vi "Allign Images.vi"(11 "subject file":path) -> (0 "shift":cluster{"left":i16, "top":i16}, 3 "picture":picture)   [LabVIEW 2013]
panel:
  in  "s":bool
  out "Intensity Graph":i16[][](graph)
  out "Array":dbl[](array[numeric])
  out "Master Picture":picture
  out "% matches":dbl
  out "max":i32
  out "rect":T1
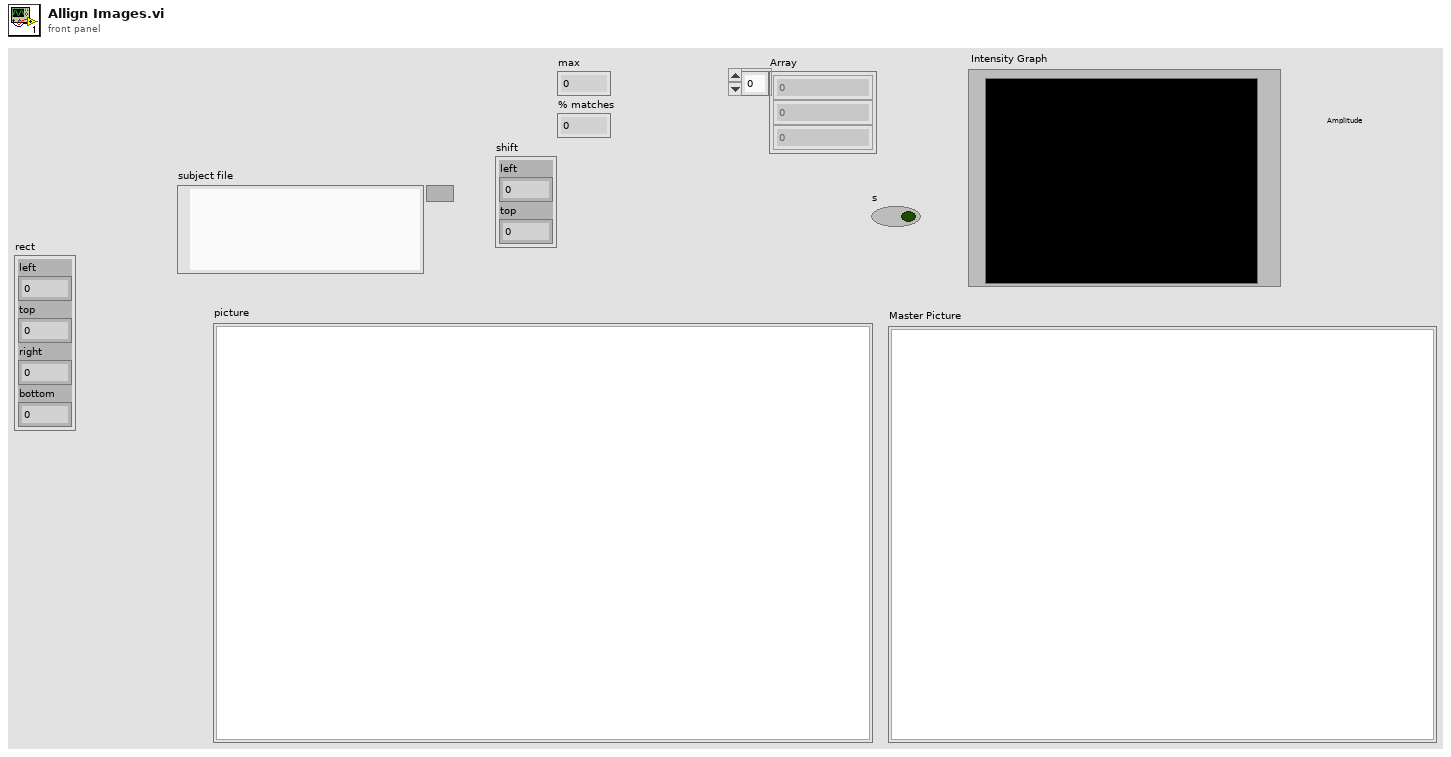
[diagram p1: front panel]
types:
  T1 = cluster{"left":i16, "top":i16, "right":i16, "bottom":i16}
  T2 = typedef "imagedata.ctl" = cluster{"image type":i32, "image depth":i32, "image":u8[], "mask":u8[], "colors":u32[], "Rectangle":cluster{"left":i16, "top":i16, "right":i16, "bottom":i16}}
  T3 = cluster{"left":i16, "top":i16, "right":i16, "bottom":i16}[]
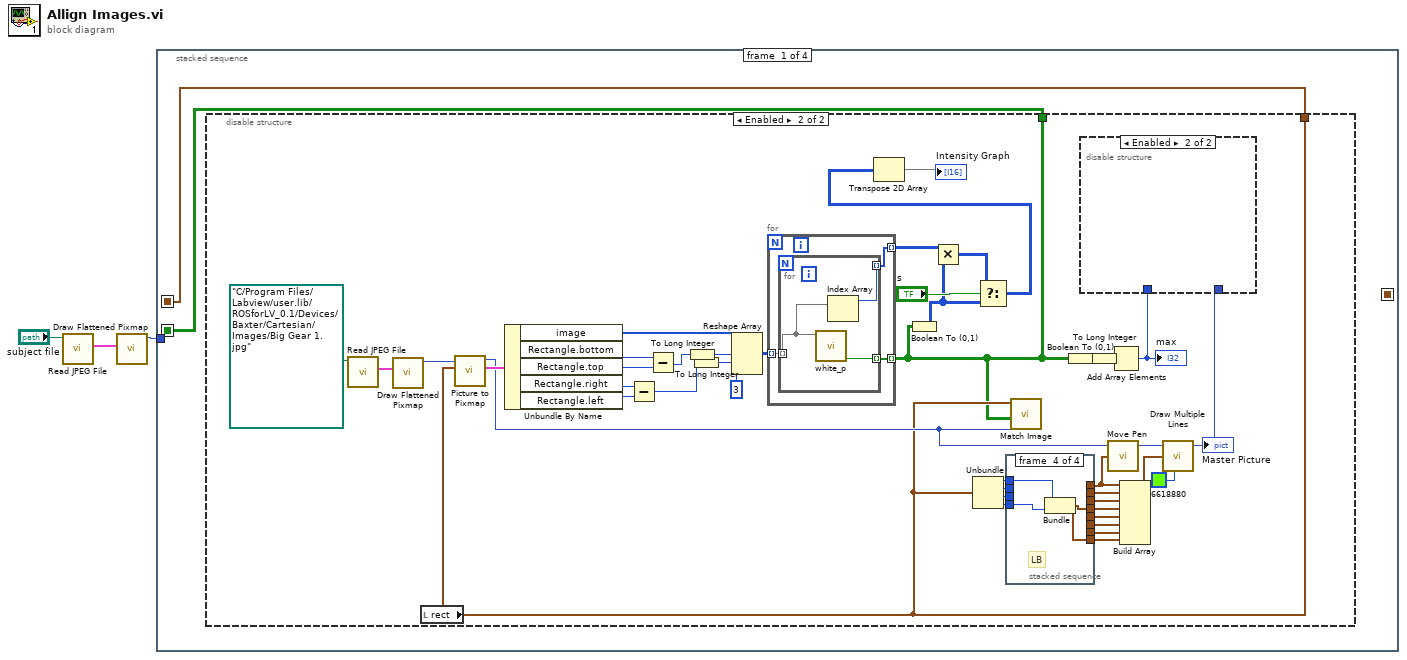
[diagram p0: block diagram]
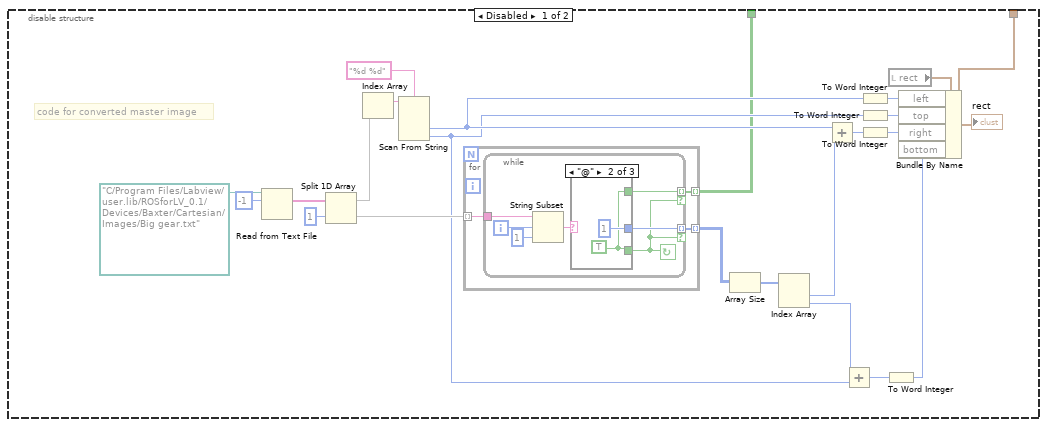
[diagram p2: hidden frame]
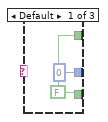
[diagram p3: hidden frame]
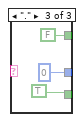
[diagram p4: hidden frame]
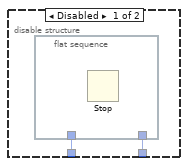
[diagram p5: hidden frame]
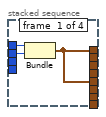
[diagram p6: hidden frame]
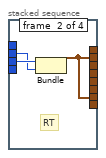
[diagram p7: hidden frame]
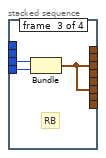
[diagram p8: hidden frame]
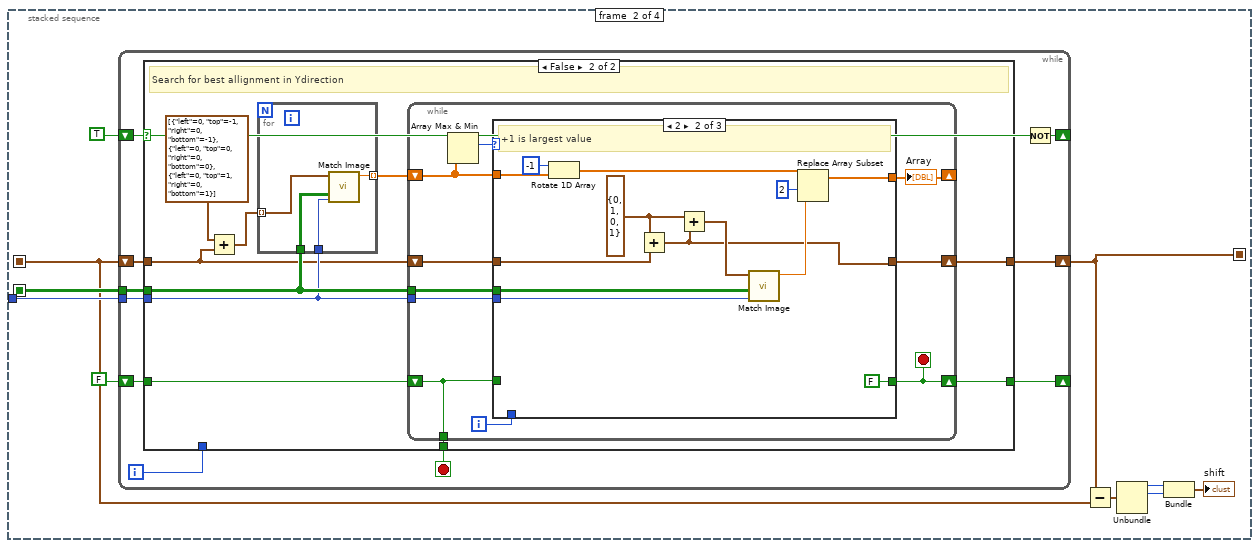
[diagram p9: hidden frame]
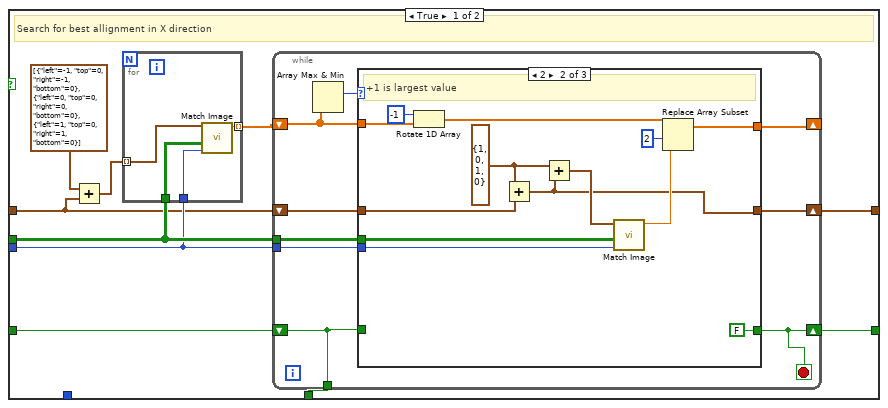
[diagram p10: hidden frame]
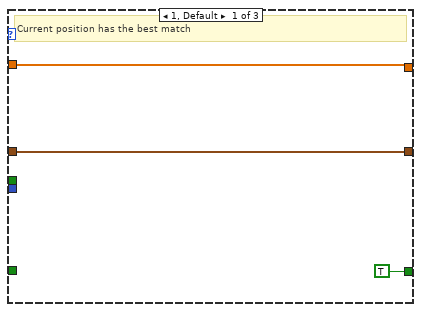
[diagram p11: hidden frame]
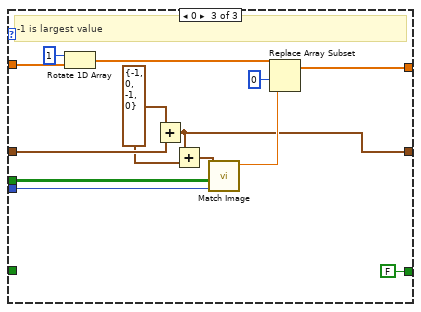
[diagram p12: hidden frame]
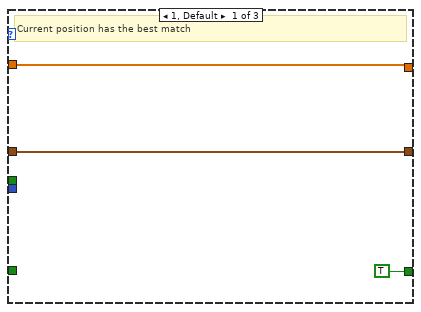
[diagram p13: hidden frame]
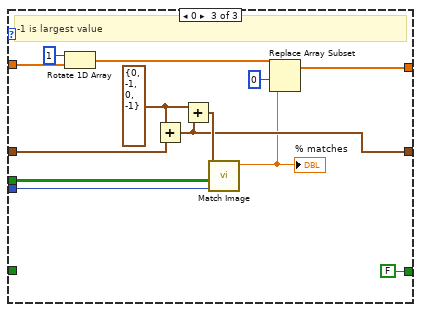
[diagram p14: hidden frame]
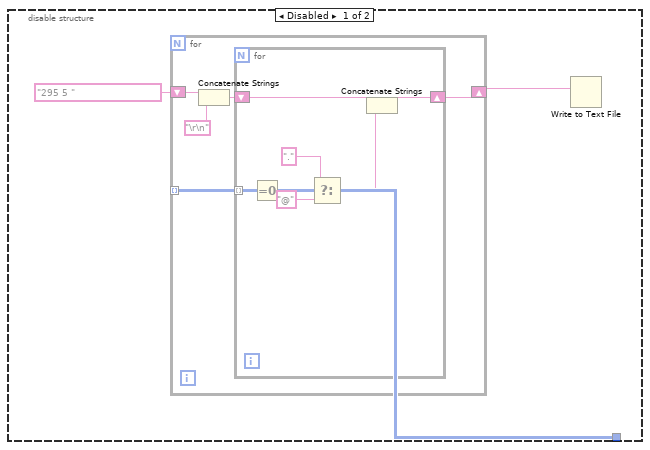
[diagram p16: hidden frame]
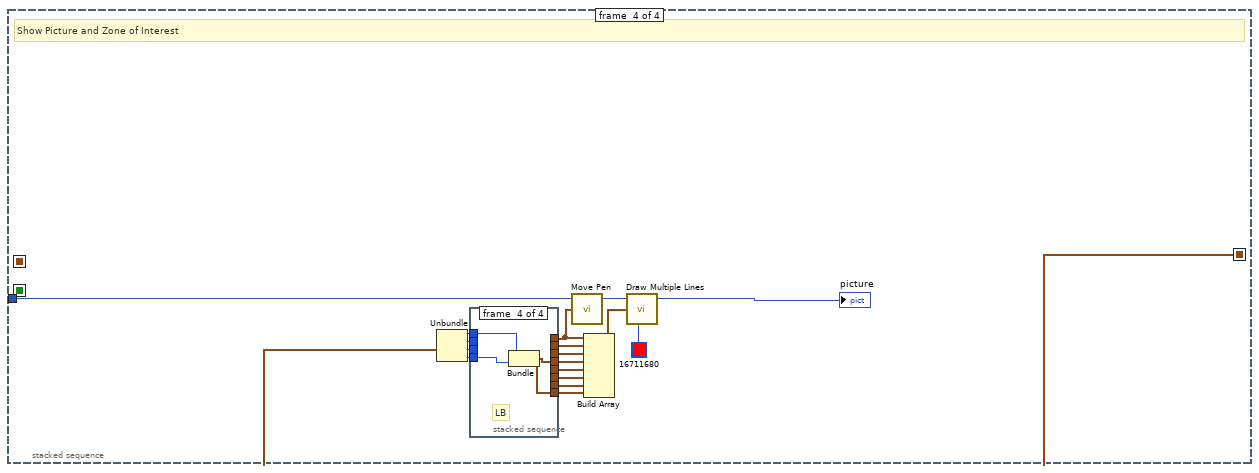
[diagram p17: hidden frame]
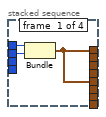
[diagram p18: hidden frame]
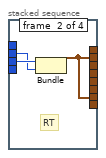
[diagram p19: hidden frame]
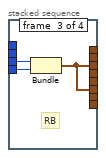
[diagram p20: hidden frame]
diagram:
  n1 = call <vilib>:"Read JPEG File.vi"("path to JPEG file"="subject file") -> ("image data"=w3:T2)  [unwired: 8 in, 2 out]
  n2 = call <vilib>:"Draw Flattened Pixmap.vi"("image data"=w3) -> ("new picture"=w2:picture)  [unwired: 8 in]
  n3 = stacked-sequence {
    seq-local: [w4 _ _ _] -> [_ w114 _ _]
    seq-local: [w5 _ _ _] -> [_ w115 _ _]
    seq-local: [_ w109 _ _] -> [_ _ _ w251]
    tunnel: w2 -> [_ w118 _ w249]
    frame #0 {
      n4 = disable-structure shown="Enabled" {
        disable-tunnel: [w8 w51] -> w5
        disable-tunnel: [w7 w71] -> w4
        frame Disabled {
          # "code for converted master image"
          n5 = Read from Text File(file (use dialog)=path "C:/Program Files/Labview/user.lib/ROSforLV_0.1/Devices/Baxter/Cartesian/Images/Big gear.txt", count=-1) -> (text=w20:string[])  [unwired: 2 in, 3 out]
          n6 = Split 1D Array(array=w20, index=1) -> (first subarray=w24:string[], second subarray=w22:string[])
          n7 = Index Array(array=w24) -> (element=w25:string)  [unwired: 1 in]
          n8 = Scan From String(format string="%d %d", input string=w25) -> (output 1=w16:i32, output 2=w15:i32)  [unwired: 4 in, 3 out]
          n9 = for {
            tunnel: [w31] -> w27 mode=indexing
            tunnel: w22 -> [w30] mode=indexing
            tunnel: [w29] -> w8 mode=indexing
            n10 = while {
              tunnel: w30 -> [w36]
              tunnel: [w34] -> w31 mode=indexing if=w32
              tunnel: [w33] -> w29 mode=indexing if=w32
              i -> [w38]
              stop <- w32 continue-if-true
              n11 = String Subset(string=w36, offset (0)=w38, length (rest)=1 ("length (rest)")) -> (substring=w35:string)
              n12 = case shown="\"@\"" w35 {
                tunnel: [w39 w41 TRUE] -> w32
                tunnel: [0 1 0] -> w34
                tunnel: [w39 w41 FALSE] -> w33
                frame Default {
                  w39 = FALSE
                }
                frame "@" {
                  w41 = TRUE
                }
                frame "." {
                }
              }
            }
          }
          n13 = Array Size(array=w27) -> (size(s)=w28:i32[])
          n14 = Index Array(array=w28) -> (element #1=w18:i32, element #2=w17:i32)  [unwired: 2 in]
          n15 = Add(x=w16, y=w18) -> (x+y=w14:i32)
          n16 = Add(x=w17, y=w15) -> (x+y=w13:i32)
          n17 = To Word Integer(number=w16) -> (16bit integer=w9:i16)
          n18 = To Word Integer(number=w15) -> (16bit integer=w10:i16)
          n19 = To Word Integer(number=w14) -> (16bit integer=w11:i16)
          n20 = To Word Integer(number=w13) -> (16bit integer=w12:i16)
          n21 = local read "rect"() -> (w6:T1)
          n22 = Bundle By Name(cluster=w6, "left"=w9, "top"=w10, "right"=w11, "bottom"=w12) -> (w7:T1)
          "rect" <- w7
        }
        frame Enabled {
          n23 = call <vilib>:"Read JPEG File.vi"("path to JPEG file"=path "C:/Program Files/Labview/user.lib/ROSforLV_0.1/Devices/Baxter/Cartesian/Images/Big Gear 1.jpg") -> ("image data"=w75:T2)  [unwired: 8 in, 2 out]
          n24 = call <vilib>:"Draw Flattened Pixmap.vi"("image data"=w75) -> ("new picture"=w73:picture)  [unwired: 8 in]
          n25 = local read "rect"() -> (w71:T1)
          n26 = call <vilib>:"Picture to Pixmap.vi"("rect"=w71, "picture"=w73) -> ("image data"=w82:T2, "new picture"=w72:picture)  [unwired: 8 in]
          n27 = Unbundle By Name(w82) -> ("image"=w79:u8[], "Rectangle.bottom"=w77:i16, "Rectangle.top"=w83:i16, "Rectangle.right"=w84:i16, "Rectangle.left"=w78:i16)
          n28 = Subtract(x=w84, y=w78) -> (x-y=w86:i16)
          n29 = Subtract(x=w77, y=w83) -> (x-y=w85:i16)
          n30 = To Long Integer(number=w85) -> (32bit integer=w87:i32)
          n31 = To Long Integer(number=w86) -> (32bit integer=w88:i32)
          n32 = Reshape Array(w79, w87, w88, 3 ("dimension size")) -> (w81:u8[][][])
          n33 = for {
            tunnel: w81 -> [w105] mode=indexing
            tunnel: [w104] -> w51 mode=indexing
            tunnel: [w103] -> w48 mode=indexing
            n34 = for {
              tunnel: w105 -> [w107] mode=indexing
              tunnel: [w108] -> w104 mode=indexing
              tunnel: [w106] -> w103 mode=indexing
              n35 = call "white_p.vi"("Array"=w107) -> ("White"=w108:bool)  [unwired: 10 in]
              n36 = Index Array(array=w107) -> (element=w106:u8)  [unwired: 1 in]
            }
          }
          n37 = Boolean To (0,1)(Boolean=w51) -> (0, 1=w47:i16[][])
          n38 = Multiply(x=w48, y=w47) -> (x*y=w46:i16[][])
          n39 = Unbundle(w71) -> ("left"=w70:i16, "top"=w69:i16, "right"=w65:i16, "bottom"=w63:i16)
          n40 = Select(t=w46, s="s", f=w47) -> (s? t:f=w50:i16[][])
          n41 = Transpose 2D Array(2D array=w50) -> (transposed array=→"Intensity Graph":i16[][])
          n42 = stacked-sequence {
            tunnel: w70 -> [w93 _ _ w102]
            tunnel: w69 -> [w92 w95 _ _]
            tunnel: [w91 _ _ _] -> w67
            tunnel: [w91 _ _ _] -> w66
            tunnel: w65 -> [_ w96 w99 _]
            tunnel: [_ w94 _ _] -> w64
            tunnel: w63 -> [_ _ w98 w101]
            tunnel: [_ _ w97 _] -> w62
            tunnel: [_ _ _ w100] -> w61
            tunnel: [_ _ w97 _] -> w54
            tunnel: [_ w94 _ _] -> w53
            tunnel: [_ _ _ w100] -> w52
            frame #0 {
              n43 = Bundle("left"=w93, "top"=w92) -> (w91:cluster{"left":i16, "top":i16})  [unwired: 1 in]
            }
            frame #1 {
              # "RT"
              n44 = Bundle("right"=w96, "top"=w95) -> (w94:cluster{"right":i16, "top":i16})  [unwired: 1 in]
            }
            frame #2 {
              # "RB"
              n45 = Bundle("right"=w99, "bottom"=w98) -> (w97:cluster{"right":i16, "bottom":i16})  [unwired: 1 in]
            }
            frame #3 {
              # "LB"
              n46 = Bundle("left"=w102, "bottom"=w101) -> (w100:cluster{"left":i16, "bottom":i16})  [unwired: 1 in]
            }
          }
          n47 = call "Match Image.vi"("picture"=w72, "Template"=w51, "rect"=w71) -> ()  [unwired: 8 in, 1 out]
          n48 = Boolean To (0,1)(Boolean=w51) -> (0, 1=w76:i16[][])
          n49 = To Long Integer(number=w76) -> (32bit integer=w56:i32[][])
          n50 = call <vilib>:"Move Pen.vi"("new position"=w67, "picture"=w72) -> ("new picture"=w68:picture)  [unwired: 3 in]
          n51 = Add Array Elements(numeric array=w56) -> (sum=w60:i32)
          "max" <- w60
          n52 = Build Array(w67, w64, w62, w61, w66, w54, w53, w52) -> (w58:cluster{"left":i16, "bottom":i16}[])
          n53 = call <vilib>:"Draw Multiple Lines.vi"("picture"=w68, "line endpoints"=w58, "color(black)"=u32 6618880) -> ("new picture"=w59:picture)  [unwired: 6 in]
          "Master Picture" <- w59
          n54 = disable-structure shown="Enabled" {
            disable-tunnel: w60 -> [w90 _]
            disable-tunnel: w59 -> [w89 _]
            frame Disabled {
              n55 = flat-sequence {
                tunnel: w90 -> [_]
                tunnel: w89 -> [_]
                frame #0 {
                  n56 = Stop() -> ()  [unwired: 1 in]
                }
              }
            }
            frame Enabled {
            }
          }
        }
      }
    }
    frame #1 {
      n57 = while {
        shift-right: [w126] -> _
        shift-left: FALSE -> [w128]
        shift-right: [w125] -> _
        shift-left: TRUE -> [w124]
        tunnel: w118 -> [w123]
        tunnel: w115 -> [w122]
        shift-right: [w120] -> w109
        shift-left: w114 -> [w121]
        i -> [w119]
        stop <- w127 stop-if-true
        n58 = case shown="False" w124 {
          tunnel: w128 -> [w138 w190]
          tunnel: [w137 w189] -> w127
          tunnel: [w136 w188] -> w126
          tunnel: w123 -> [w134 w186]
          tunnel: w122 -> [w135 w187]
          tunnel: w121 -> [w131 w183]
          tunnel: [w129 w181] -> w120
          tunnel: w119 -> [_ _]
          frame True {
            # "Search for best allignment in X direction"
            n59 = Add(x=T3 [{"left"=-1, "top"=0, "right"=-1, "bottom"=0}, {"left"=0, "top"=0, "right"=0, "bottom"=0}, {"left"=1, "top"=0, "right"=1, "bottom"=0}], y=w131) -> (x+y=w130:T3)
            n60 = for {
              tunnel: w135 -> [w142]
              tunnel: w134 -> [w141]
              tunnel: [w140] -> w133 mode=indexing
              tunnel: w130 -> [w139] mode=indexing
              n61 = call "Match Image.vi"("picture"=w141, "Template"=w142, "rect"=w139) -> ("%"=w140:dbl)  [unwired: 8 in]
            }
            n62 = while {
              shift-right: [w150] -> w136
              shift-left: w138 -> [w149]
              tunnel: [w149] -> w137
              tunnel: w134 -> [w147]
              tunnel: w135 -> [w146]
              shift-right: [w144] -> _
              shift-left: w133 -> [w148]
              shift-right: [w143] -> w129
              shift-left: w131 -> [w145]
              stop <- w150 stop-if-true
              n63 = Array Max & Min(array=w148) -> (max index (indices)=w151:i32)  [unwired: 3 out]
              n64 = case shown="2" w151 {
                tunnel: w149 -> [_ _ _]
                tunnel: [TRUE FALSE FALSE] -> w150
                tunnel: w148 -> [w153 w166 w179]
                tunnel: w147 -> [_ w164 w177]
                tunnel: w146 -> [_ w163 w176]
                tunnel: w145 -> [w152 w162 w175]
                tunnel: [w153 w158 w171] -> w144
                tunnel: [w152 w155 w170] -> w143
                frame 1, Default {
                  # "Current position has the best match"
                }
                frame 2 {
                  w156 = T1 {"left"=1, "top"=0, "right"=1, "bottom"=0} ("rect")
                  # "+1 is largest value"
                  n65 = Rotate 1D Array(1:w166, 2:-1 ("n")) -> (0:w161:dbl[])
                  n66 = Add(x=w156, y=w162) -> (x+y=w155:T1)
                  n67 = Add(x=w156, y=w155) -> (x+y=w157:T1)
                  n68 = call "Match Image.vi"("picture"=w164, "Template"=w163, "rect"=w157) -> ("%"=w160:dbl)  [unwired: 8 in]
                  n69 = Replace Array Subset(array=w161, new element=w160, index=2) -> (w158:dbl[])
                }
                frame 0 {
                  w169 = T1 {"left"=-1, "top"=0, "right"=-1, "bottom"=0} ("rect")
                  # "-1 is largest value"
                  n70 = Rotate 1D Array(1:w179, 2:1 ("n")) -> (0:w174:dbl[])
                  n71 = Add(x=w169, y=w175) -> (x+y=w170:T1)
                  n72 = Add(x=w170, y=w169) -> (x+y=w168:T1)
                  n73 = call "Match Image.vi"("picture"=w177, "Template"=w176, "rect"=w168) -> ("%"=w173:dbl)  [unwired: 8 in]
                  n74 = Replace Array Subset(array=w174, new element=w173, index=0) -> (w171:dbl[])
                }
              }
            }
          }
          frame False {
            # "Search for best allignment in Ydirection"
            n75 = Add(x=T3 [{"left"=0, "top"=-1, "right"=0, "bottom"=-1}, {"left"=0, "top"=0, "right"=0, "bottom"=0}, {"left"=0, "top"=1, "right"=0, "bottom"=1}], y=w183) -> (x+y=w182:T3)
            n76 = for {
              tunnel: w187 -> [w194]
              tunnel: w186 -> [w193]
              tunnel: [w192] -> w185 mode=indexing
              tunnel: w182 -> [w191] mode=indexing
              n77 = call "Match Image.vi"("picture"=w193, "Template"=w194, "rect"=w191) -> ("%"=w192:dbl)  [unwired: 8 in]
            }
            n78 = while {
              shift-right: [w203] -> w188
              shift-left: w190 -> [w202]
              tunnel: [w202] -> w189
              tunnel: w186 -> [w200]
              tunnel: w187 -> [w199]
              shift-right: [w197] -> _
              shift-left: w185 -> [w201]
              shift-right: [w196] -> w181
              shift-left: w183 -> [w198]
              i -> [w195]
              stop <- w203 stop-if-true
              n79 = Array Max & Min(array=w201) -> (max index (indices)=w204:i32)  [unwired: 3 out]
              n80 = case shown="2" w204 {
                tunnel: w202 -> [_ _ _]
                tunnel: [TRUE FALSE FALSE] -> w203
                tunnel: w201 -> [w206 w219 w232]
                tunnel: w200 -> [_ w217 w230]
                tunnel: w199 -> [_ w216 w229]
                tunnel: w198 -> [w205 w215 w228]
                tunnel: [w206 w211 w225] -> w197
                tunnel: [w205 w208 w222] -> w196
                tunnel: w195 -> [_ _ _]
                frame 1, Default {
                  # "Current position has the best match"
                }
                frame 2 {
                  w209 = T1 {"left"=0, "top"=1, "right"=0, "bottom"=1} ("rect")
                  # "+1 is largest value"
                  n81 = Rotate 1D Array(1:w219, 2:-1 ("n")) -> (0:w214:dbl[])
                  n82 = Add(x=w209, y=w215) -> (x+y=w208:T1)
                  n83 = Add(x=w209, y=w208) -> (x+y=w210:T1)
                  n84 = call "Match Image.vi"("picture"=w217, "Template"=w216, "rect"=w210) -> ("%"=w213:dbl)  [unwired: 8 in]
                  n85 = Replace Array Subset(array=w214, new element=w213, index=2) -> (w211:dbl[])
                }
                frame 0 {
                  w223 = T1 {"left"=0, "top"=-1, "right"=0, "bottom"=-1} ("rect")
                  # "-1 is largest value"
                  n86 = Rotate 1D Array(1:w232, 2:1 ("n")) -> (0:w227:dbl[])
                  n87 = Add(x=w223, y=w228) -> (x+y=w222:T1)
                  n88 = Add(x=w223, y=w222) -> (x+y=w224:T1)
                  n89 = call "Match Image.vi"("picture"=w230, "Template"=w229, "rect"=w224) -> ("%"=w221:dbl)  [unwired: 8 in]
                  "% matches" <- w221
                  n90 = Replace Array Subset(array=w227, new element=w221, index=0) -> (w225:dbl[])
                }
              }
              "Array" <- w197
            }
          }
        }
        n91 = Not(x=w124) -> (.not. x?=w125:bool)
      }
      n92 = Subtract(x=w109, y=w114) -> (x-y=w113:T1)
      n93 = Unbundle(w113) -> ("left"=w112:i16, "top"=w111:i16)  [unwired: 2 out]
      n94 = Bundle("left"=w112, "top"=w111) -> (→"shift":cluster{"left":i16, "top":i16})  [unwired: 1 in]
    }
    frame #2 {
      n95 = disable-structure shown="Enabled" {
        disable-tunnel: _ -> [w236 _]
        frame Disabled {
          n96 = for {
            tunnel: w236 -> [w241] mode=indexing
            shift-right: [w238] -> w234
            shift-left: "295 5 " -> [w239]
            n97 = Concatenate Strings(w239, "\r\n") -> (w240:string)
            n98 = for {
              tunnel: w241 -> [w248] mode=indexing
              shift-right: [w242] -> w238
              shift-left: w240 -> [w243]
              n99 = Equal To 0?(x=w248) -> (x = 0?=w247:bool)
              n100 = Select(t=".", s=w247, f="@") -> (s? t:f=w244:string)
              n101 = Concatenate Strings(w243, w244) -> (w242:string)
            }
          }
          n102 = Write to Text File(text=w234) -> ()  [unwired: 3 in, 3 out]
        }
        frame Enabled {
        }
      }
    }
    frame #3 {
      # "Show Picture and Zone of Interest"
      n103 = Unbundle(w251) -> ("left"=w266:i16, "top"=w265:i16, "right"=w261:i16, "bottom"=w259:i16)
      n104 = stacked-sequence {
        tunnel: w266 -> [w269 _ _ w278]
        tunnel: w265 -> [w268 w271 _ _]
        tunnel: [w267 _ _ _] -> w263
        tunnel: [w267 _ _ _] -> w262
        tunnel: w261 -> [_ w272 w275 _]
        tunnel: [_ w270 _ _] -> w260
        tunnel: w259 -> [_ _ w274 w277]
        tunnel: [_ _ w273 _] -> w258
        tunnel: [_ _ _ w276] -> w257
        tunnel: [_ _ w273 _] -> w254
        tunnel: [_ w270 _ _] -> w253
        tunnel: [_ _ _ w276] -> w252
        frame #0 {
          n105 = Bundle("left"=w269, "top"=w268) -> (w267:cluster{"left":i16, "top":i16})  [unwired: 1 in]
        }
        frame #1 {
          # "RT"
          n106 = Bundle("right"=w272, "top"=w271) -> (w270:cluster{"right":i16, "top":i16})  [unwired: 1 in]
        }
        frame #2 {
          # "RB"
          n107 = Bundle("right"=w275, "bottom"=w274) -> (w273:cluster{"right":i16, "bottom":i16})  [unwired: 1 in]
        }
        frame #3 {
          # "LB"
          n108 = Bundle("left"=w278, "bottom"=w277) -> (w276:cluster{"left":i16, "bottom":i16})  [unwired: 1 in]
        }
      }
      n109 = call <vilib>:"Move Pen.vi"("new position"=w263, "picture"=w249) -> ("new picture"=w264:picture)  [unwired: 3 in]
      n110 = Build Array(w263, w260, w258, w257, w262, w254, w253, w252) -> (w256:cluster{"left":i16, "bottom":i16}[])
      n111 = call <vilib>:"Draw Multiple Lines.vi"("picture"=w264, "line endpoints"=w256, "color(black)"=u32 16711680) -> ("new picture"=→"picture":picture)  [unwired: 6 in]
    }
  }
